vi "SystemChangeEvtCallback.vi"(4 "SystemStateChange":refnum<user-event>, 5 "Event Data":cluster{"state":u8}, 6 "Control Ref":T1, 7 "Event Common Data":T2) -> ()   [LabVIEW 2020, in "NI_VS Workspace ExecutionAPI.lvlib"]
uses:
  <vilib>/NI VeriStand/Execution/Workspace/NI_VS Workspace ExecutionAPI.lvlib
  <vilib>/NI VeriStand/Execution/Workspace/WorkspaceAPI.ctl
  NationalInstruments.VeriStand.ClientAPI
  <vilib>/NI VeriStand/Execution/Workspace/SystemStateEvent.ctl
  <vilib>/Utility/VariantDataType/VariantType.lvlib
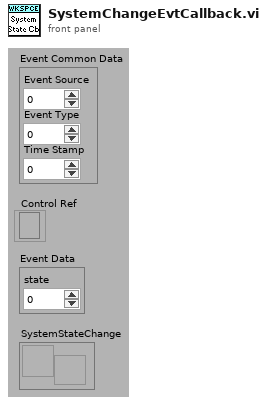
[diagram p1: front panel]
types:
  T1 = typedef "NI_VS Workspace ExecutionAPI.lvlib/WorkspaceAPI.ctl" = refnum<k24>
  T2 = cluster{"Event Source":i32, "Event Type":u32, "Time Stamp":u32}
  T3 = typedef "NI_VS Workspace ExecutionAPI.lvlib/SystemStateEvent.ctl" = enum16{"Stop Configuration", "Start Configuration", "Shut Down"}
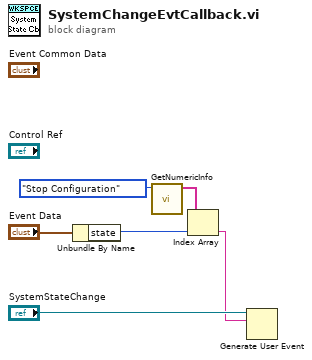
[diagram p0: block diagram]
diagram:
  n1 = Unbundle By Name("Event Data") -> ("state"=w3:u8)
  n2 = call <vilib>:"GetNumericInfo.vi"("Variant"=SystemStateEvent."Stop Configuration" ("SystemState")) -> ("EnumNames"=w2:string[])  [unwired: 1 in, 9 out]
  n3 = Index Array(array=w2, index=w3) -> (element=w1:string)
  n4 = Generate User Event(user event="SystemStateChange", event data cluster=w1) -> ()  [unwired: 2 in, 2 out]
